vi "WaitFor(abort).vi"(1 "config":refnum<queue>, 4 "Wait For Chamber":bool, 5 "Timeout":dbl, 6 "Wait For Position":bool, 7 "Delay":dbl, 8 "Wait For Field":bool, 9 "Wait For Temperature":bool, 10 "error in (no error)":errorcluster, 11 "Instrument Ref In":refnum<k24>) -> (2 "error out":errorcluster, 3 "Instrument Ref Out":refnum<k24>)   [LabVIEW 2019, in "SubVI.lvlib"]
uses:
  SubVI.lvlib
  lib/QDInstrument.dll
  config.ctl
  Instance           2 15Saved   WaitFor .vi
  Instance           1 15Saved   WaitFor .vi
panel:
  # "(真是通道1，假是通道2)"
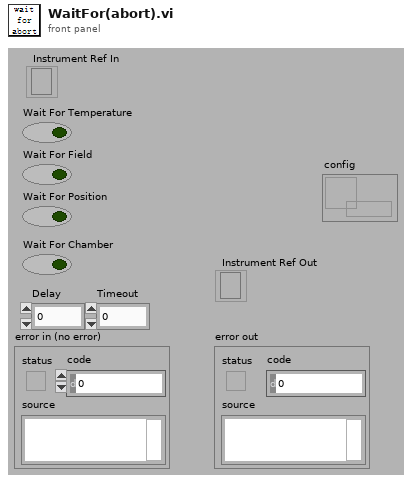
[diagram p1: front panel]
types:
  T1 = typedef "config.ctl" = cluster{"error":bool, "initialize":string, "数值":dbl, "6221":cluster{"6221 Resource":refnum<visa-resource-name>, "Delta status":bool}, "7001":cluster{"Ch":bool}}
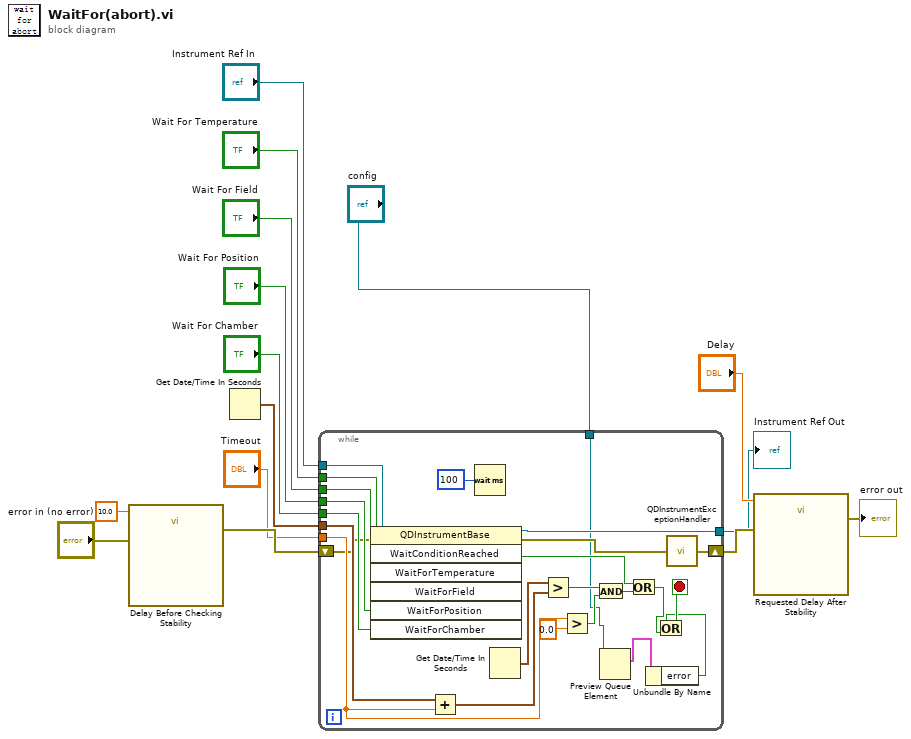
[diagram p0: block diagram]
diagram:
  n1 = call "Delay Before Checking Stability"("error in (no error)"="error in (no error)", "Delay Time (s)"=10.0) -> ("error out"=w6:errorcluster)  [unwired: 9 in]
  n2 = Get Date/Time In Seconds() -> (seconds since 1Jan1904=w5:timestamp)
  n3 = while {
    shift-right: [w21] -> w11
    shift-left: w6 -> [w24]
    tunnel: "Wait For Temperature" -> [w28]
    tunnel: "Wait For Field" -> [w27]
    tunnel: "Wait For Position" -> [w26]
    tunnel: "Wait For Chamber" -> [w25]
    tunnel: w5 -> [w38]
    tunnel: "Timeout" -> [w35]
    tunnel: "Instrument Ref In" -> [w30]
    tunnel: [w29] -> w2
    tunnel: "config" -> [w20]
    stop <- w18 stop-if-true
    n4 = invoke class="QDInstrumentBase" method="WaitConditionReached"(reference=w30, error in=w24, "WaitForTemperature"=w28, "WaitForField"=w27, "WaitForPosition"=w26, "WaitForChamber"=w25) -> (reference out=w29:refnum<k24>, error out=w22:errorcluster, "WaitConditionReached"=w23:bool)  [unwired: 1 in, 4 out]
    n5 = Add(x=w38, y=w35) -> (x+y=w36:timestamp)
    n6 = Wait (ms)(milliseconds to wait=u32 100) -> ()  [unwired: 1 out]
    n7 = Get Date/Time In Seconds() -> (seconds since 1Jan1904=w37:timestamp)
    n8 = Greater?(x=w37, y=w36) -> (0:w33:bool)
    n9 = Greater?(x=w35, y=0.0) -> (0:w32:bool)
    n10 = And(x=w33, y=w32) -> (x .and. y?=w31:bool)
    n11 = Preview Queue Element(queue=w20) -> (element=w17:T1)  [unwired: 2 in, 3 out]
    n12 = Or(x=w23, y=w31) -> (x .or. y?=w19:bool)
    n13 = Unbundle By Name(w17) -> ("error"=w16:bool)
    n14 = Or(x=w16, y=w19) -> (x .or. y?=w18:bool)
    n15 = call "QDInstrumentExceptionHandler.vi"("Error in"=w22) -> ("Error out"=w21:errorcluster)
  }
  "Instrument Ref Out" <- w2
  n16 = call "Requested Delay After Stability"("error in (no error)"=w11, "Delay Time (s)"="Delay") -> ("error out"=→"error out":errorcluster)  [unwired: 9 in]
